vi "updateMDF_Z.vi"(7 "MDF":T1(array[cluster]), 8 "index":i32, 10 "buoy Y":i32, 11 "buoy X":i32) -> (2 "OthersideY":i32, 3 "OthersideX":i32, 5 "MDF out":T1(array[cluster]))   [LabVIEW 2014]
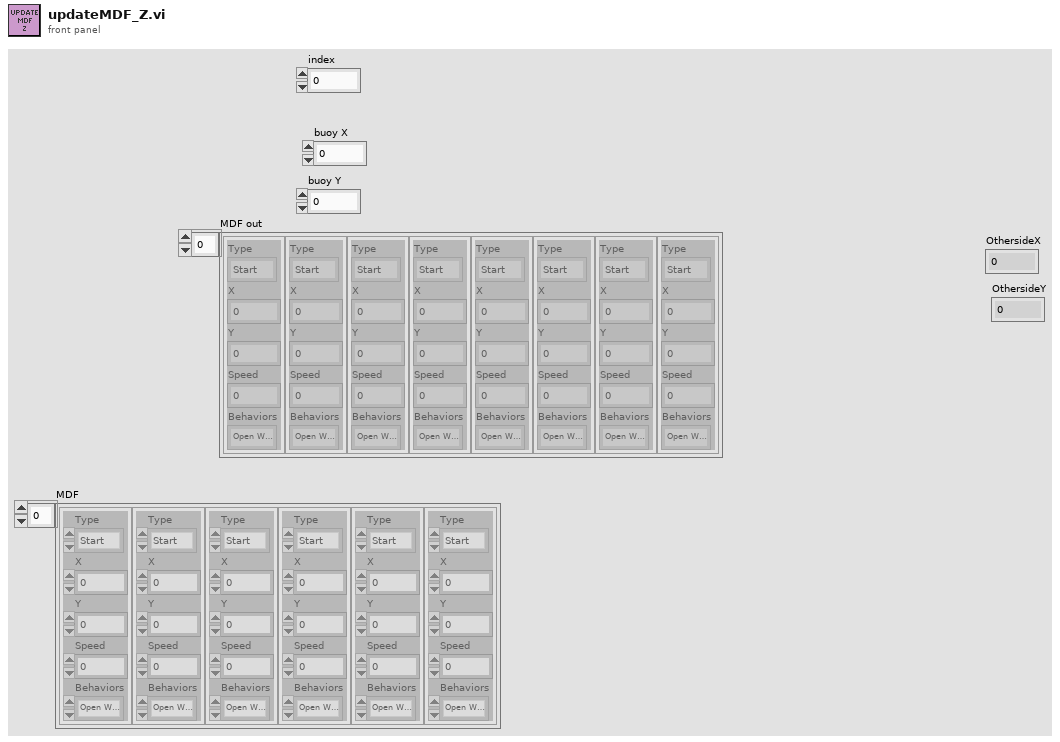
[diagram p1: front panel]
types:
  T1 = cluster{"Type":enum16{"Start", "Buoy Circling", "Waypoint", "End"}, "X":i32, "Y":i32, "Speed":i32, "Behaviors":enum16{"Open Water Transit", "P-Wall Follow", "S-Wall Follow", "Get Unstuck"}}[]
  T2 = enum16{"Open Water Transit", "P-Wall Follow", "S-Wall Follow", "Get Unstuck"}
  T3 = cluster{"Type":enum16{"Start", "Buoy Circling", "Waypoint", "End"}, "X":i32, "Y":i32, "Speed":i32, "Behaviors":enum16{"Open Water Transit", "P-Wall Follow", "S-Wall Follow", "Get Unstuck"}}
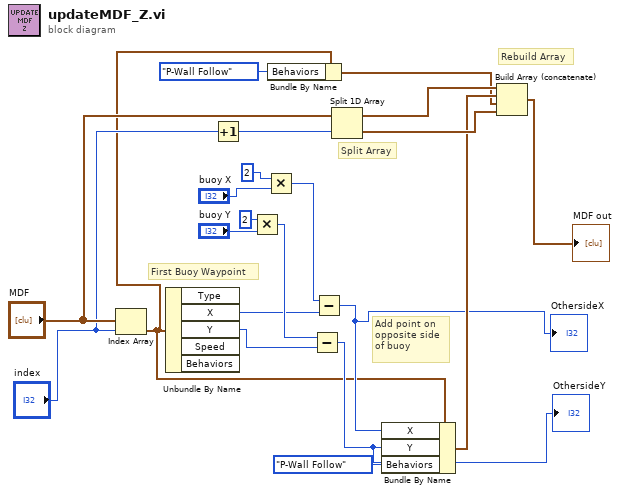
[diagram p0: block diagram]
diagram:
  # "First Buoy Waypoint"
  # "Add point on \nopposite side \nof buoy"
  # "Rebuild Array"
  # "Split Array"
  n1 = Index Array(array="MDF", index="index") -> (element=w5:T3)
  n2 = Unbundle By Name(w5) -> ("X"=w4:i32, "Y"=w3:i32)  [unwired: 3 out]
  n3 = Increment(x="index") -> (x+1=w10:i32)
  n4 = Multiply(x=2, y="buoy Y") -> (x*y=w16:i32)
  n5 = Multiply(x=2, y="buoy X") -> (x*y=w19:i32)
  n6 = Bundle By Name(cluster=w5, "Behaviors"=T2."P-Wall Follow") -> (w1:T3)
  n7 = Subtract(x=w16, y=w3) -> (x-y=w7:i32)
  "OthersideY" <- w7
  n8 = Subtract(x=w19, y=w4) -> (x-y=w8:i32)
  "OthersideX" <- w8
  n9 = Split 1D Array(array="MDF", index=w10) -> (first subarray=w15:T1, second subarray=w14:T1)
  n10 = Bundle By Name(cluster=w5, "X"=w8, "Y"=w7, "Behaviors"=T2."P-Wall Follow") -> (w12:T3)
  n11 = Build Array (concatenate)(w15, w12, w1, w14) -> (→"MDF out":T1)
